vi "Update Buffer.vi"(4 "Buffer (ms)":u32, 5 "Data Points mode":bool, 6 "T0 (s)":u32, 7 "Graph style":string(combo)="Chart", 8 "Times to add":u32[](array[numeric]), 9 "Values to add":dbl[](array[numeric]), 10 "Times (in)":u32[](array[numeric]), 11 "Graph (in)":dbl[](array[numeric])) -> (2 "Times (out)":u32[](array[numeric]), 3 "Graph (out)":dbl[](array[numeric]))   [LabVIEW 2009]
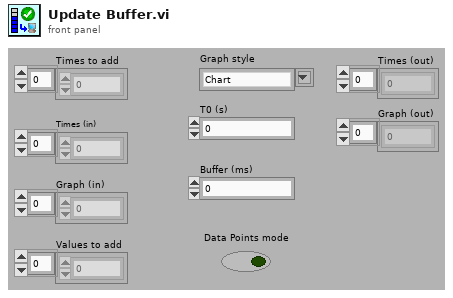
[diagram p1: front panel]
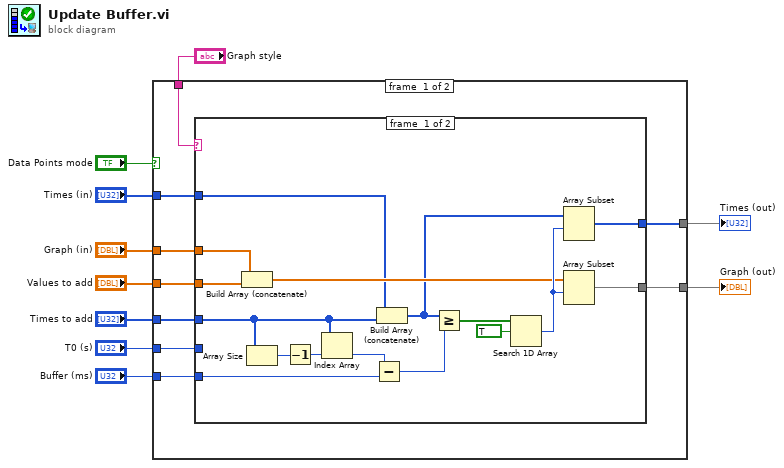
[diagram p0: block diagram]
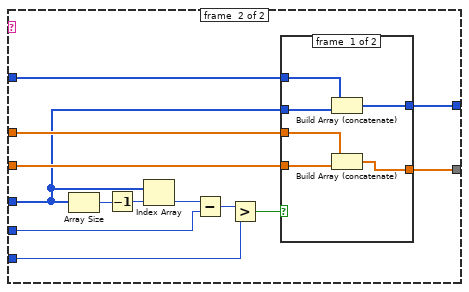
[diagram p2: hidden frame]
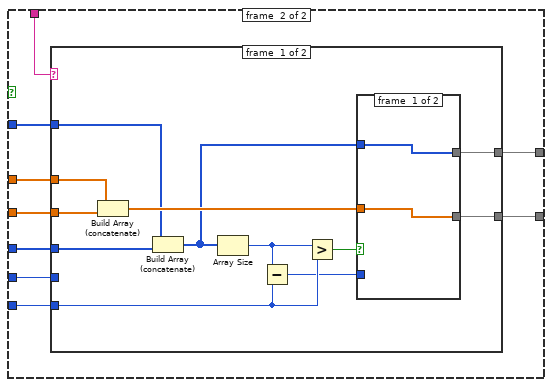
[diagram p4: hidden frame]
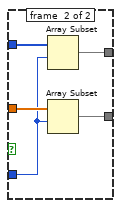
[diagram p5: hidden frame]
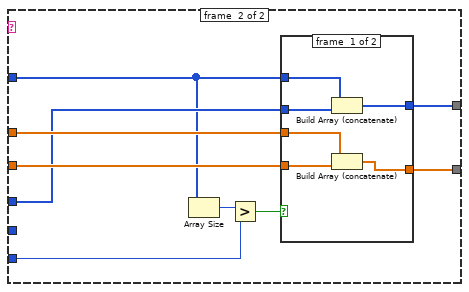
[diagram p6: hidden frame]
diagram:
  n1 = case shown="True" "Data Points mode" {
    tunnel: "Buffer (ms)" -> [w19 w65]
    tunnel: "T0 (s)" -> [w18 w64]
    tunnel: "Graph (in)" -> [w17 w63]
    tunnel: "Times (in)" -> [w16 w62]
    tunnel: [w15 w61] -> w6
    tunnel: [w14 w60] -> w5
    tunnel: "Graph style" -> [w13 w59]
    tunnel: "Values to add" -> [w12 w58]
    tunnel: "Times to add" -> [w11 w57]
    frame #0 {
      n2 = case shown="\"Chart\", Default" w13 {
        tunnel: [w31 w46] -> w14
        tunnel: [w30 w44] -> w15
        tunnel: w12 -> [w29 w45]
        tunnel: w16 -> [w26 w43]
        tunnel: w17 -> [w25 w42]
        tunnel: w18 -> [_ w41]
        tunnel: w19 -> [w24 w40]
        tunnel: w11 -> [w21 w36]
        frame #0 {
          n3 = Build Array (concatenate)(w25, w29) -> (w28:dbl[])
          n4 = Array Size(array=w21) -> (size(s)=w23:i32)
          n5 = Decrement(x=w23) -> (x-1=w22:i32)
          n6 = Index Array(array=w21, index=w22) -> (element=w20:u32)
          n7 = Subtract(x=w20, y=w24) -> (x-y=w35:u32)
          n8 = Build Array (concatenate)(w26, w21) -> (w27:u32[])
          n9 = Greater Or Equal?(x=w27, y=w35) -> (x >= y?=w34:bool[])
          n10 = Search 1D Array(1D array=w34, element=TRUE) -> (index of element=w32:i32)  [unwired: 1 in]
          n11 = Array Subset(array=w27, index=w32) -> (w31:u32[])  [unwired: 1 in]
          n12 = Array Subset(array=w28, index=w32) -> (w30:dbl[])  [unwired: 1 in]
        }
        frame #1 {
          n13 = Array Size(array=w36) -> (size(s)=w39:i32)
          n14 = Decrement(x=w39) -> (x-1=w38:i32)
          n15 = Index Array(array=w36, index=w38) -> (element=w37:u32)
          n16 = Subtract(x=w37, y=w41) -> (x-y=w48:u32)
          n17 = Greater?(x=w48, y=w40) -> (0:w47:bool)
          n18 = case shown="False" w47 {
            tunnel: w36 -> [w54 _]
            tunnel: [w53 w56] -> w46
            tunnel: w45 -> [w52 _]
            tunnel: [w51 w55] -> w44
            tunnel: w43 -> [w50 w56]
            tunnel: w42 -> [w49 w55]
            frame #0 {
              n19 = Build Array (concatenate)(w50, w54) -> (w53:u32[])
              n20 = Build Array (concatenate)(w49, w52) -> (w51:dbl[])
            }
            frame #1 {
            }
          }
        }
      }
    }
    frame #1 {
      n21 = case shown="\"Chart\", Default" w59 {
        tunnel: [w77 w92] -> w60
        tunnel: [w76 w90] -> w61
        tunnel: w58 -> [w75 w91]
        tunnel: w62 -> [w73 w85]
        tunnel: w63 -> [w72 w89]
        tunnel: w64 -> [_ _]
        tunnel: w65 -> [w67 w88]
        tunnel: w57 -> [w71 w87]
        frame #0 {
          n22 = Build Array (concatenate)(w72, w75) -> (w74:dbl[])
          n23 = Build Array (concatenate)(w73, w71) -> (w70:u32[])
          n24 = Array Size(array=w70) -> (size(s)=w68:i32)
          n25 = Subtract(x=w68, y=w67) -> (x-y=w66:u32)
          n26 = Greater?(x=w68, y=w67) -> (0:w69:bool)
          n27 = case shown="True" w69 {
            tunnel: [w79 w84] -> w77
            tunnel: [w78 w83] -> w76
            tunnel: w74 -> [w78 w82]
            tunnel: w70 -> [w79 w81]
            tunnel: w66 -> [_ w80]
            frame #0 {
            }
            frame #1 {
              n28 = Array Subset(array=w81, index=w80) -> (w84:u32[])  [unwired: 1 in]
              n29 = Array Subset(array=w82, index=w80) -> (w83:dbl[])  [unwired: 1 in]
            }
          }
        }
        frame #1 {
          n30 = Array Size(array=w85) -> (size(s)=w86:i32)
          n31 = Greater?(x=w86, y=w88) -> (0:w93:bool)
          n32 = case shown="False" w93 {
            tunnel: w87 -> [w99 _]
            tunnel: [w98 w101] -> w92
            tunnel: w91 -> [w97 _]
            tunnel: [w96 w100] -> w90
            tunnel: w85 -> [w95 w101]
            tunnel: w89 -> [w94 w100]
            frame #0 {
              n33 = Build Array (concatenate)(w95, w99) -> (w98:u32[])
              n34 = Build Array (concatenate)(w94, w97) -> (w96:dbl[])
            }
            frame #1 {
            }
          }
        }
      }
    }
  }
  "Graph (out)" <- w6
  "Times (out)" <- w5
